vi "MB Ethernet Slave Demon - Single Port - Single Connection.vi"(6 "Period":u32=200) -> ()   [LabVIEW 2011]
uses:
  <vilib>/Platform/TimedLoop/XDataNode/timing_clust.ctl
  <vilib>/Platform/TimedLoop/XDataNode/nitl_modes.ctl
  <vilib>/Platform/TimedLoop/XDataNode/wakeup.ctl
  MB Globals.vi
  <vilib>/Platform/TimedLoop/XDataNode/XDataNode.xnode
  <vilib>/Platform/TimedLoop/XDataNode/XDNodeRunTimeDep.lvlib
panel:
  in  "Timeout":i32=5000
  in  "Port":u16=502
  out "Demon Running":bool
  # "VI Name: MB Ethernet Slave Demon.vi\nPurpose: Modbus Demon"
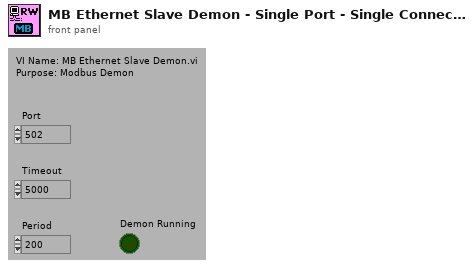
[diagram p1: front panel]
types:
  T1 = typedef "XDNodeRunTimeDep.lvlib/timing_clust.ctl" = cluster{"Expected End [f-1]":u64, "Actual End [f-1]":u64, "Finished Late? [f-1]":bool, "Expected End [i-1]":u64, "Actual End [i-1]":u64, "Finished Late? [i-1]":bool, "Expected Start [i]":u64, "Actual Start [i]":u64, "Expected Start [f]":u64, "Actual Start [f]":u64, "Source Name":string, "Structure Name":string, "Period":i64, "Deadline":i64, "Offset":i64, "Start":i64, "Priority":i32, "Timeout":i32, "Mode":T2, "Wakeup Reason":T3, "Error":errorcluster, "Source Type":string, "Secondary Source Type":string, "Global End Time":u64, "Global Start Time":u64, "Frame Duration":u64, "Iteration Duration":u64, "Assigned CPU":i32, "I/O Scan Engine Mode":u32}
  T2 = typedef "XDNodeRunTimeDep.lvlib/nitl_modes.ctl" = enum32{"No Change", "Process missed periods, maintain original phase", "Discard missed periods, maintain original phase", "Process missed periods, ignore original phase", "Discard missed periods, ignore original phase"}
  T3 = typedef "XDNodeRunTimeDep.lvlib/wakeup.ctl" = enum32{"Normal", "Aborted", "Asynchronous wakeup", "Timing source error", "Timed loop error", "Timeout"}
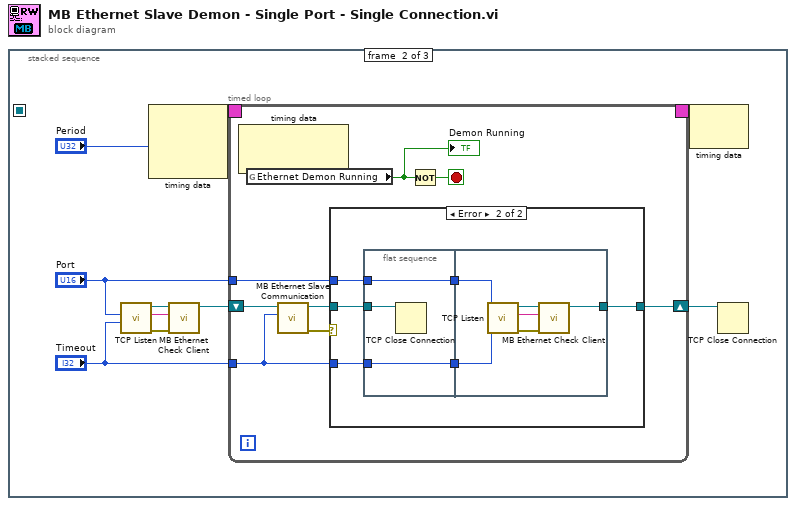
[diagram p0: block diagram]
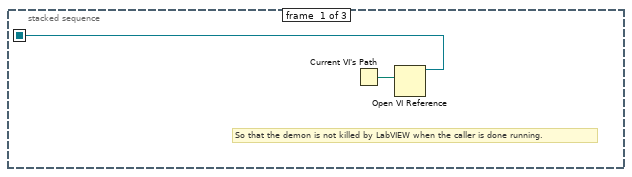
[diagram p2: hidden frame]
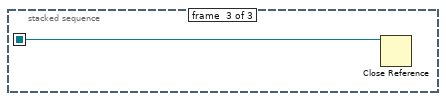
[diagram p4: hidden frame]
diagram:
  n1 = stacked-sequence {
    seq-local: [w1 _ _] -> [_ _ w43]
    frame #0 {
      # "So that the demon is not killed by LabVIEW when the caller is done running."
      n2 = Current VI's Path() -> (path=w2:path)
      n3 = Open VI Reference(vi path=w2) -> (vi reference=w1:refnum<vi>)  [unwired: 1 in, 5 out]
    }
    frame #1 {
      n4 = call <vilib>:"TCP Listen.vi"("timeout ms (wait forever: -1)"="Timeout", "port"="Port") -> ("error out"=w8:errorcluster, "remote address"=w6:string, "connection ID"=w9:refnum<k5>)  [unwired: 2 in, 5 out]
      n5 = node-c288("Period") -> (w3:T1)  [unwired: 2 out]
      n6 = call "MB Ethernet Check Client.vi"("error in (no error)"=w8, "Remote Address"=w6, "Connection ID in"=w9) -> ("Connection ID out"=w7:refnum<k5>)  [unwired: 8 out]
      n7 = timed-loop {
        tunnel: "Port" -> [w14]
        shift-left: w7 -> [w18]
        shift-right: [w16] -> w11
        tunnel: "Timeout" -> [w15]
        timing-out: [_] -> w4
        timing: w3 -> [_]
        stop <- w20 stop-if-true
        n8 = node-c288() -> ()  [unwired: 3 out]
        n9 = global read "MB Globals.vi" "Ethernet Demon Running"() -> (w19:bool)
        "Demon Running" <- w19
        n10 = call "MB Ethernet Slave Communication.vi"("Timeout"=w15, "Connection ID"=w18) -> ("error out"=w17:errorcluster, "Connection ID (dup)"=w13:refnum<k5>)  [unwired: 1 in, 7 out]
        n11 = case shown="Error" w17 {
          tunnel: [w22 w23] -> w16
          tunnel: w15 -> [_ w25]
          tunnel: w14 -> [_ w27]
          tunnel: w13 -> [w22 w28]
          frame No Error {
          }
          frame Error {
            n12 = flat-sequence {
              tunnel: w28 -> [w31]
              tunnel: w27 -> [w30]
              tunnel: [w30] -> w26
              tunnel: w25 -> [w29]
              tunnel: [w29] -> w24
              tunnel: w26 -> [w37]
              tunnel: w24 -> [w36]
              tunnel: [w34] -> w23
              frame #0 {
                n13 = TCP Close Connection(connection ID=w31) -> ()  [unwired: 1 in, 3 out]
              }
              frame #1 {
                n14 = call <vilib>:"TCP Listen.vi"("timeout ms (wait forever: -1)"=w36, "port"=w37) -> ("error out"=w33:errorcluster, "remote address"=w32:string, "connection ID"=w35:refnum<k5>)  [unwired: 2 in, 5 out]
                n15 = call "MB Ethernet Check Client.vi"("error in (no error)"=w33, "Remote Address"=w32, "Connection ID in"=w35) -> ("Connection ID out"=w34:refnum<k5>)  [unwired: 8 out]
              }
            }
          }
        }
        n16 = Not(x=w19) -> (.not. x?=w20:bool)
      }
      n17 = node-c288(w4) -> ()  [unwired: 1 out]
      n18 = TCP Close Connection(connection ID=w11) -> ()  [unwired: 1 in, 3 out]
    }
    frame #2 {
      n19 = Close Reference(reference=w43) -> ()  [unwired: 1 in, 1 out]
    }
  }
